vi "BMU诊断标定.vi"(8 "CAN端口":u16(ring), 9 "设备索引号":u16(ring), 10 "CAN卡类型":u32(ring)=21) -> ()   [LabVIEW 2013] (continued)
              n52 = call <vilib>:"Get Key Names.vi"("section"=w374, "refnum"=w373) -> ("key names"=w175:string[], "refnum out"=w375:T19)  [unwired: 6 in, 2 out]
              n53 = for {
                tunnel: w375 -> [w387]
                tunnel: w374 -> [w386]
                tunnel: w175 -> [w385] mode=indexing
                tunnel: [w384] -> w174 mode=indexing
                n54 = call-poly <vilib>:"Read Key.vi"("section"=w386, "key"=w385, "refnum"=w387) -> ("value"=w384:string)  [unwired: 5 in, 3 out]
              }
              n55 = Search 1D Array(1D array=w175, element="总电压过高一级" ("元素"), start index (0)=0 ("开始索引(0)")) -> (index of element=w255:i32)
              n56 = Search 1D Array(1D array=w175, element="风机开启温度" ("元素"), start index (0)=w255) -> (index of element=w246:i32)
              n57 = Search 1D Array(1D array=w175, element="电池串联" ("元素"), start index (0)=w246) -> (index of element=w244:i32)
              n58 = Decrement(x=w255) -> (x-1=w372:i32)
              n59 = Array Subset(array=w175, index=1 ("索引"), length=w372) -> (w220:string[])
              n60 = Array Subset(array=w174, index=1 ("索引"), length=w372) -> (w217:string[])
              n61 = Delete From Array(array=w217, length=7 ("长度"), index=0 ("索引")) -> (deleted portion=w214:string[], array with subset deleted=w164:string[])
              n62 = Delete From Array(array=w220, length=7 ("长度"), index=0 ("索引")) -> (array with subset deleted=w173:string[])  [unwired: 1 out]
              n63 = Search 1D Array(1D array=w175, element="分流器型号" ("元素")) -> (index of element=w178:i32)  [unwired: 1 in]
              n64 = Index Array(array=w174, index=0 ("索引")) -> (element=w348:string)
              n65 = Decimal String To Number(string=w348) -> (number=w165:i32)  [unwired: 2 in, 1 out]
              n66 = Search 1D Array(1D array=w173, element="主板电池节数" ("元素")) -> (index of element=w339:i32)  [unwired: 1 in]
              n67 = Search 1D Array(1D array=w173, element="主板温度起始值" ("元素")) -> (index of element=w336:i32)  [unwired: 1 in]
              n68 = Search 1D Array(1D array=w173, element="第一个保险通道" ("元素")) -> (index of element=w335:i32)  [unwired: 1 in]
              n69 = Search 1D Array(1D array=w173, element="主板温度个数" ("元素")) -> (index of element=w337:i32)  [unwired: 1 in]
              n70 = Search 1D Array(1D array=w173, element="主板电压起始值" ("元素")) -> (index of element=w338:i32)  [unwired: 1 in]
              n71 = Search 1D Array(1D array=w173, element="第1通道电压个数" ("元素")) -> (index of element=w334:i32)  [unwired: 1 in]
              n72 = Index Array(array=w174, index=w178) -> (element=w177:string)
              n73 = for {
                N: 4 -> [_]
                tunnel: w214 -> [w383] mode=indexing
                tunnel: [w382] -> w363 mode=indexing
                n74 = Fract/Exp String To Number(string=w383) -> (number=w382:dbl)  [unwired: 3 in, 1 out]
              }
              n75 = Increment(x=w165) -> (x+1=w347:i32)
              n76 = Increment(x=w165) -> (x+1=w332:i32)
              n77 = Increment(x=w165) -> (x+1=w345:i32)
              n78 = Increment(x=w165) -> (x+1=w346:i32)
              n79 = global write "读配置文件全局.vi" "从板个数"(w165) -> ()
              n80 = local write "从板个数"(w165) -> ()
              n81 = Decimal String To Number(string=w177) -> (number=w176:i32)  [unwired: 2 in, 1 out]
              n82 = Index Array(array=w214, index #1=4 ("索引"), index #2=5 ("索引"), index #3=6 ("索引")) -> (element #1=w354:string, element #2=w353:string, element #3=w352:string)
              n83 = Index Array(array=w363) -> (element #1=w361:dbl, element #2=w360:dbl, element #3=w359:dbl, element #4=w358:dbl)  [unwired: 4 in]
              n84 = global write "EV05全局变量1.vi" "分流器型号"(w176) -> ()
              n85 = Array Subset(array=w164, index=w339, length=w347) -> (w331:string[])
              n86 = Array Subset(array=w164, index=w338, length=w346) -> (w329:string[])
              n87 = Array Subset(array=w164, index=w337, length=w345) -> (w328:string[])
              n88 = Array Subset(array=w164, index=w336, length=w332) -> (w327:string[])
              n89 = Array Subset(array=w164, index=w335, length=20 ("长度")) -> (w326:string[])
              n90 = Array Subset(array=w164, index=w334, length=w333) -> (w330:string[])
              n91 = Multiply(x=w165, y=2) -> (x*y=w166:i32)
              n92 = control-ref of="项目信息2"() -> (w366:refnum<vi>)
              n93 = Array Subset(array=w164, index=0 ("索引"), length=w166) -> (w163:string[])
              n94 = Insert Into Array(array=w331, new element #1=w330, new element #2=w329, new element #3=w328, new element #4=w327, new element #5=w326) -> ()  [unwired: 1 in, 1 out]
              n95 = property class="Clust (严格)"(reference=w366) -> (reference out=w364:refnum<vi>, "Value"=w365:T9)  [unwired: 1 in, 1 out]
              n96 = Multiply(x=w165, y=2) -> (x*y=w170:i32)
              n97 = Array Subset(array=w173, index=w339, length=w332) -> (w204:string[])
              n98 = Array Subset(array=w173, index=w338, length=w332) -> (w202:string[])
              n99 = Array Subset(array=w173, index=w337, length=w332) -> (w201:string[])
              n100 = Array Subset(array=w173, index=w336) -> (w200:string[])  [unwired: 1 in]
              n101 = Array Subset(array=w173, index=w335, length=w333) -> (w199:string[])
              n102 = Array Subset(array=w173, index=w334, length=w333) -> (w203:string[])
              n103 = Array Subset(array=w173, index=0 ("索引"), length=w170) -> (w169:string[])
              n104 = global write "读配置文件全局.vi" "表格输入"(w163) -> ()
              n105 = Build Array(w169, w163) -> (w325:string[][])
              n106 = Bundle(cluster=w365, "电池额定容量(A)"=w361, "使用者"=w351, "电池实际容量(A)"=w360, "车架(牌)号"=w353, "配置文件版本"=w352, "SOH(%)"=w358, "SOC(%)"=w359, "产品编号"=w354) -> (w191:T9)  [unwired: 1 in]
              n107 = Transpose 2D Array(2D array=w325) -> (transposed array=w192:string[][])
              n108 = Multiply(x=w165, y=4) -> (x*y=w196:i32)
              n109 = Insert Into Array(array=w204, new element #1=w203, new element #2=w202, new element #3=w201, new element #4=w200, new element #5=w199) -> (w198:string[])  [unwired: 1 in]
              n110 = Add(x=w196, y=44) -> (x+y=w194:i32)
              n111 = local write "项目信息"(w192) -> ()
              n112 = property class="Clust (严格)"(reference=w364, "Value"=w191) -> ()  [unwired: 1 in, 2 out]
              n113 = global write "读配置文件全局.vi" "项目信息"(w191) -> ()
              n114 = Array Subset(array=w174, index=w244, length=15 ("长度")) -> (w182:string[])
              n115 = Array Subset(array=w198, index=0 ("索引"), length=w194) -> ()  [unwired: 1 out]
              n116 = Array Subset(array=w174, index=w246, length=15 ("长度")) -> (w251:string[])
              n117 = Delete From Array(array=w182, length=4 ("长度"), index=6 ("索引")) -> (deleted portion=w238:string[], array with subset deleted=w237:string[])
              n118 = for {
                tunnel: w251 -> [w379] mode=indexing
                tunnel: [w378] -> w250 mode=indexing
                n119 = Fract/Exp String To Number(string=w379) -> (number=w378:dbl)  [unwired: 3 in, 1 out]
              }
              n120 = for {
                tunnel: w237 -> [w377] mode=indexing
                tunnel: [w376] -> w236 mode=indexing
                n121 = Fract/Exp String To Number(string=w377) -> (number=w376:dbl)  [unwired: 3 in, 1 out]
              }
              n122 = Array Subset(array=w174, index=w255, length=51 ("长度")) -> (w324:string[])
              n123 = for {
                tunnel: w324 -> [w381] mode=indexing
                tunnel: [w380] -> w323 mode=indexing
                n124 = Fract/Exp String To Number(string=w381) -> (number=w380:dbl)  [unwired: 3 in, 1 out]
              }
              n125 = Index Array(array=w236) -> (element #1=w231:dbl, element #2=w230:dbl, element #3=w229:dbl, element #4=w228:dbl, element #5=w227:dbl, element #6=w226:dbl, element #7=w225:dbl, element #8=w224:dbl, element #9=w223:dbl, element #10=w222:dbl, element #11=w221:dbl)  [unwired: 11 in]
              n126 = Delete From Array(array=w250, length=7 ("长度"), index=0 ("索引")) -> (deleted portion=w187:dbl[], array with subset deleted=w248:dbl[])
              n127 = Delete From Array(array=w323, length=17 ("长度"), index=0 ("索引")) -> (deleted portion=w184:dbl[], array with subset deleted=w320:dbl[])
              n128 = Array To Cluster(array=w187) -> (cluster=w249:T20)
              n129 = global write "读配置文件全局.vi" "加热控制参数"(w187) -> ()
              n130 = Index Array(array=w248) -> (element #1=w212:dbl, element #2=w211:dbl, element #3=w210:dbl, element #4=w209:dbl, element #5=w208:dbl, element #6=w207:dbl, element #7=w206:dbl, element #8=w205:dbl)  [unwired: 8 in]
              n131 = Delete From Array(array=w320, length=17 ("长度"), index=0 ("索引")) -> (deleted portion=w183:dbl[], array with subset deleted=w180:dbl[])
              n132 = Index Array(array=w238) -> (element #1=w235:string, element #2=w234:string, element #3=w232:string, element #4=w233:string)  [unwired: 4 in]
              n133 = local write "加热控制参数"(w249) -> ()
              n134 = global write "读配置文件全局.vi" "一级故障"(w184) -> ()
              n135 = local read "一级故障 5"() -> (w213:T12)
              n136 = control-ref of="电池信息"() -> (w242:refnum<vi>)
              n137 = global write "读配置文件全局.vi" "二级故障"(w183) -> ()
              n138 = global write "读配置文件全局.vi" "三级故障"(w180) -> ()
              n139 = Bundle(cluster=w213, "最大允许单体电压"=w212, "最大允许总电压"=w208, "最小允许单体电压"=w211, "最大允许充电电流"=w210, "最小允许充电电流"=w209, "最大允许充电温度"=w207, "最小允许充电温度"=w206, "电流步长"=w205) -> (w186:T12)
              n140 = property class="Clust (严格)"(reference=w242) -> (reference out=w243:refnum<vi>, "Value"=w241:T13)  [unwired: 1 in, 1 out]
              n141 = Bundle(cluster=w241, "电池串联"=w231, "电池并联"=w230, "累计放电总安时"=w224, "电池包额定容量"=w229, "电池包额定能量(kWh)"=w228, "电池包额定总电压"=w227, "累计充电总安时"=w225, "电池充满次数"=w222, "电池放空次数"=w223, "电池充电次数"=w221, "电池生产日期"=w232, "电池厂家"=w235, "电池类型"=w234, "电池包组号"=w233, "实际容量"=w226) -> (w181:T13)  [unwired: 2 in]
              n142 = Cluster To Array(cluster=w186) -> (array=w185:dbl[])
              n143 = local write "一级故障 5"(w186) -> ()
              n144 = global write "读配置文件全局.vi" "充电控制参数"(w185) -> ()
              n145 = Index Array(array=w184) -> (element #1=w313:dbl, element #2=w312:dbl, element #3=w311:dbl, element #4=w310:dbl, element #5=w309:dbl, element #6=w308:dbl, element #7=w307:dbl, element #8=w306:dbl, element #9=w305:dbl, element #10=w304:dbl, element #11=w303:dbl, element #12=w302:dbl, element #13=w301:dbl, element #14=w300:dbl, element #15=w299:dbl, element #16=w298:dbl, element #17=w297:dbl)  [unwired: 17 in]
              n146 = global write "读配置文件全局.vi" "电池信息"(w181) -> ()
              n147 = Index Array(array=w183) -> (element #1=w280:dbl, element #2=w281:dbl, element #3=w282:dbl, element #4=w283:dbl, element #5=w284:dbl, element #6=w285:dbl, element #7=w286:dbl, element #8=w287:dbl, element #9=w288:dbl, element #10=w289:dbl, element #11=w290:dbl, element #12=w291:dbl, element #13=w292:dbl, element #14=w293:dbl, element #15=w294:dbl, element #16=w295:dbl, element #17=w296:dbl)  [unwired: 17 in]
              n148 = Index Array(array=w180) -> (element #1=w275:dbl, element #2=w274:dbl, element #3=w273:dbl, element #4=w272:dbl, element #5=w271:dbl, element #6=w270:dbl, element #7=w269:dbl, element #8=w268:dbl, element #9=w267:dbl, element #10=w266:dbl, element #11=w265:dbl, element #12=w264:dbl, element #13=w263:dbl, element #14=w262:dbl, element #15=w261:dbl, element #16=w260:dbl, element #17=w259:dbl)  [unwired: 17 in]
              n149 = control-ref of="一级故障 3"() -> (w258:refnum<vi>)
              n150 = control-ref of="一级故障 2"() -> (w277:refnum<vi>)
              n151 = property class="Clust (严格)"(reference=w277) -> (reference out=w279:refnum<vi>, "Value"=w278:T10)  [unwired: 1 in, 1 out]
              n152 = property class="Clust (严格)"(reference=w258) -> (reference out=w257:refnum<vi>, "Value"=w276:T10)  [unwired: 1 in, 1 out]
              n153 = property class="Clust (严格)"(reference=w243, "Value"=w181) -> ()  [unwired: 1 in, 2 out]
              n154 = Bundle(cluster=w278, "总电压过高"=w280, "整组电压不均衡"=w284, "SOC过高"=w292, "单体电压过高"=w288, "总电压过低"=w281, "温度过高"=w282, "温度过低"=w283, "单组电压不均衡"=w285, "整组温度不均衡"=w286, "单组温度不均衡"=w287, "单体电压过低"=w289, "充电电流过高"=w290, "放电电流过高"=w291, "SOC过低"=w293, "内阻过大"=w294, "极柱温度过高"=w295, "SOH过低"=w296) -> (w189:T10)
              n155 = Bundle(cluster=w276, "总电压过高"=w275, "整组电压不均衡"=w271, "SOC过高"=w263, "单体电压过高"=w267, "总电压过低"=w274, "温度过高"=w273, "温度过低"=w272, "单组电压不均衡"=w270, "整组温度不均衡"=w269, "单组温度不均衡"=w268, "单体电压过低"=w266, "充电电流过高"=w265, "放电电流过高"=w264, "SOC过低"=w262, "内阻过大"=w261, "极柱温度过高"=w260, "SOH过低"=w259) -> (w188:T10)
              n156 = control-ref of="一级故障"() -> (w316:refnum<vi>)
              n157 = property class="Clust (严格)"(reference=w316) -> (reference out=w314:refnum<vi>, "Value"=w315:T10)  [unwired: 1 in, 1 out]
              n158 = Bundle(cluster=w315, "总电压过高"=w313, "整组电压不均衡"=w309, "SOC过高"=w301, "单体电压过高"=w305, "总电压过低"=w312, "温度过高"=w311, "温度过低"=w310, "单组电压不均衡"=w308, "整组温度不均衡"=w307, "单组温度不均衡"=w306, "单体电压过低"=w304, "充电电流过高"=w303, "放电电流过高"=w302, "SOC过低"=w300, "内阻过大"=w299, "极柱温度过高"=w298, "SOH过低"=w297) -> (w190:T10)
              n159 = property class="Clust (严格)"(reference=w314, "Value"=w190) -> ()  [unwired: 1 in, 2 out]
              n160 = property class="Clust (严格)"(reference=w279, "Value"=w189) -> ()  [unwired: 1 in, 2 out]
              n161 = property class="Clust (严格)"(reference=w257, "Value"=w188) -> ()  [unwired: 1 in, 2 out]
            }
            frame #2 {
              w452 = 1 ("索引")
              # "均衡计算-电压高阀值1级"
              n162 = call <vilib>:"Get Section Names.vi"("refnum"=w467) -> ("section names"=w468:string[], "refnum out"=w472:T19)  [unwired: 8 in, 1 out]
              n163 = Delete From Array(array=w468, length=2 ("长度"), index=0 ("索引")) -> (array with subset deleted=w471:string[])  [unwired: 1 out]
              n164 = for {
                tunnel: w471 -> [w488] mode=indexing
                tunnel: w472 -> [w489]
                tunnel: [w481] -> w450 mode=indexing
                tunnel: [w480] -> w394
                n165 = call <vilib>:"Get Key Names.vi"("section"=w488, "refnum"=w489) -> ("key names"=w480:string[], "refnum out"=w487:T19)  [unwired: 6 in, 2 out]
                n166 = for {
                  tunnel: w480 -> [w493] mode=indexing
                  tunnel: w488 -> [w492]
                  tunnel: w487 -> [w491]
                  tunnel: [w490] -> w481 mode=indexing
                  n167 = call-poly <vilib>:"Read Key.vi"("section"=w492, "key"=w493, "refnum"=w491) -> ("value"=w490:string)  [unwired: 5 in, 3 out]
                }
                n168 = Index Array(array=w481, index=0 ("索引")) -> (element=w484:string)
                n169 = local read "输出数组"() -> (w485:string[][])
                n170 = Decimal String To Number(string=w484) -> (number=w483:i32)  [unwired: 2 in, 1 out]
                n171 = Decrement(x=w483) -> (x-1=w479:i32)
                n172 = Replace Array Subset(array=w485, new element=w481, index (col)=w479) -> (w482:string[][])  [unwired: 1 in]
                n173 = local write "输出数组"(w482) -> ()
              }
              "key names" <- w394
              n174 = Decrement(x=w388) -> (x-1=w466:i32)
              n175 = Index Array(array=w450, index (row)=w466) -> (element=w393:string[])  [unwired: 1 in]
              n176 = Search 1D Array(1D array=w394, element="风机开启温度" ("元素")) -> (index of element=w455:i32)  [unwired: 1 in]
              n177 = Search 1D Array(1D array=w394, element="电压过高一级" ("元素"), start index (0)=w455) -> (index of element=w419:i32)
              n178 = Search 1D Array(1D array=w394, element="均衡计算-电压高阀值1级" ("元素"), start index (0)=w419) -> (index of element=w417:i32)
              n179 = Array Subset(array=w393, index=w417, length=17 ("长度")) -> (w416:string[])
              n180 = Decrement(x=w455) -> (x-1=w453:i32)
              n181 = Array Subset(array=w393, index=w452, length=w453) -> (w391:string[])
              n182 = Array Subset(array=w393, index=w419, length=21 ("长度")) -> (w464:string[])
              n183 = Array Subset(array=w394, index=w452, length=w453) -> (w430:string[])
              n184 = Index Array(array=w393, index=0 ("索引")) -> (element=w425:string)
              n185 = Array Subset(array=w393, index=w455, length=7 ("长度")) -> (w458:string[])
              n186 = for {
                tunnel: w416 -> [w474] mode=indexing
                tunnel: [w473] -> w415 mode=indexing
                n187 = Fract/Exp String To Number(string=w474) -> (number=w473:dbl)  [unwired: 3 in, 1 out]
              }
              n188 = for {
                tunnel: w464 -> [w476] mode=indexing
                tunnel: [w475] -> w465 mode=indexing
                n189 = Fract/Exp String To Number(string=w476) -> (number=w475:dbl)  [unwired: 3 in, 1 out]
              }
              n190 = Decimal String To Number(string=w425) -> (number=w424:i32)  [unwired: 2 in, 1 out]
              n191 = for {
                tunnel: w458 -> [w478] mode=indexing
                tunnel: [w477] -> w427 mode=indexing
                n192 = Fract/Exp String To Number(string=w478) -> (number=w477:dbl)  [unwired: 3 in, 1 out]
              }
              n193 = global write "读配置文件全局2.vi" "从板板号"(w424) -> ()
              n194 = Delete From Array(array=w465, length=7 ("长度"), index=0 ("索引")) -> (deleted portion=w429:dbl[], array with subset deleted=w461:dbl[])
              n195 = Array To Cluster(array=w427) -> (cluster=w449:T20)
              n196 = global write "读配置文件全局2.vi" "加热控制参数"(w427) -> ()
              n197 = Delete From Array(array=w461, length=7 ("长度"), index=0 ("索引")) -> (deleted portion=w422:dbl[], array with subset deleted=w423:dbl[])
              n198 = local write "加热控制参数"(w449) -> ()
              n199 = Array To Cluster(array=w429) -> (cluster=w433:T20)
              n200 = Array To Cluster(array=w423) -> (cluster=w431:T20)
              n201 = Array To Cluster(array=w422) -> (cluster=w432:T20)
              n202 = local write "从板号"(w388) -> ()
              n203 = global write "读配置文件全局2.vi" "三级故障阀值"(w423) -> ()
              n204 = global write "读配置文件全局2.vi" "一级故障阀值"(w429) -> ()
              n205 = global write "读配置文件全局2.vi" "二级故障阀值"(w422) -> ()
              n206 = local write "一级故障 6"(w433) -> ()
              n207 = local write "一级故障 8"(w431) -> ()
              n208 = local write "一级故障 7"(w432) -> ()
              n209 = Search 1D Array(1D array=w430, element="第1通道电压个数" ("元素")) -> (index of element=w441:i32)  [unwired: 1 in]
              n210 = Search 1D Array(1D array=w430, element="电压个数" ("元素")) -> ()  [unwired: 1 in, 1 out]
              n211 = Search 1D Array(1D array=w430, element="温度个数" ("元素")) -> (index of element=w443:i32)  [unwired: 1 in]
              n212 = Search 1D Array(1D array=w430, element="第一个保险通道" ("元素")) -> (index of element=w442:i32)  [unwired: 1 in]
              n213 = Array Subset(array=w391, length=2 ("长度")) -> (w438:string[])  [unwired: 1 in]
              n214 = Array Subset(array=w391, index=w443, length=2 ("长度")) -> (w436:string[])
              n215 = Array Subset(array=w391, index=w442, length=20 ("长度")) -> (w435:string[])
              n216 = Array Subset(array=w391, index=w441, length=20 ("长度")) -> (w437:string[])
              n217 = Array Subset(array=w391, length=27 ("长度")) -> (w390:string[])  [unwired: 1 in]
              n218 = Insert Into Array(array=w438, new element #1=w437, new element #2=w436, new element #3=w435) -> ()  [unwired: 1 in, 1 out]
              n219 = Build Array(string[] ["电压个数", "温度个数", "第一个保险通道", "第一个保险位置", "第二个保险通道", "第二个保险位置", "第三个保险通道", "第三个保险位置", "第四个保险通道", "第四个保险位置", "第五个保险通道", "第五个保险位置", "第六个保险通道", "第六个保险位置", "第七个保险通道", "第七个保险位置", "第八个保险通道", "第八个保险位置", "第九个保险通道", "第九个保险位置", "第十个保险通道", "第十个保险位置", "第1通道电压个数", "第2通道电压个数", "第3通道电压个数", "第4通道电压个数", "第5通道电压个数"], w390) -> (w434:string[][])
              n220 = global write "读配置文件全局2.vi" "表格"(w390) -> ()
              n221 = Index Array(array=w415) -> (element #1=w412:dbl, element #2=w411:dbl, element #3=w410:dbl, element #4=w409:dbl, element #5=w408:dbl, element #6=w407:dbl, element #7=w406:dbl, element #8=w405:dbl, element #9=w404:dbl, element #10=w403:dbl, element #11=w402:dbl, element #12=w401:dbl, element #13=w400:dbl, element #14=w399:dbl, element #15=w398:dbl, element #16=w397:dbl, element #17=w396:dbl, element #18=w395:dbl)  [unwired: 18 in]
              n222 = Transpose 2D Array(2D array=w434) -> (transposed array=w428:string[][])
              n223 = local write "项目信息 2"(w428) -> ()
              n224 = local read "均衡参数"() -> (w414:T17)
              n225 = Bundle(cluster=w414, "充电结束电压(90%)"=w405, "充电结束电压(91%)"=w404, "充电结束电压(92%)"=w403, "充电结束电压(93%)"=w402, "充电结束电压(94%)"=w401, "均衡计算-电压高阀值1级"=w412, "均衡计算-电压高阀值2级"=w411, "均衡计算-电压低阀值1级"=w410, "均衡计算-电压低阀值2级"=w409, "均衡计算-最低电压阀值"=w408, "均衡停止-最低电压阀值"=w407, "均衡计算-电压极差阀值"=w406, "充电结束电压(95%)"=w400, "充电结束电压(96%)"=w399, "充电结束电压(97%)"=w398, "充电结束电压(98%)"=w397, "充电结束电压(99%)"=w396, "充电结束电压(100%)"=w395) -> (w413:T17)
              n226 = local write "均衡参数"(w413) -> ()
            }
            frame #3 {
              n227 = Build Array("读取完成") -> (w497:string[])
              n228 = property on="全部写入" class="Bool (严格)"("DisabledEnum"=0) -> ()  [unwired: 2 in, 2 out]
              n229 = call "表格编辑.vi"("新元素/子数组"=w497, "活动单元格:单元格背景色"=u32 6618880, "MCListbox引用句柄"=w494) -> ()  [unwired: 9 out]
            }
          }
        }
      }
    }
  }
  n230 = local write "项目信息 2"(string[][] [["电压个数", "36"], ["温度个数", "45"], ["第一个保险通道", "0"], ["第一个保险位置", "0"], ["第二个保险通道", "0"], ["第二个保险位置", "0"], ["第三个保险通道", "0"], ["第三个保险位置", "0"], ["第四个保险通道", "0"], ["第四个保险位置", "0"], ["第五个保险通道", "0"], ["第五个保险位置", "0"], ["第六个保险通道", "0"], ["第六个保险位置", "0"], ["第七个保险通道", "0"], ["第七个保险位置", "0"], ["第八个保险通道", "0"], ["第八个保险位置", "0"], ["第九个保险通道", "0"], ["第九个保险位置", "0"], ["第十个保险通道", "0"], ["第十个保险位置", "0"], ["第1通道电压个数", "11"], ["第2通道电压个数", "12"], ["第3通道电压个数", "12"], ["第4通道电压个数", "12"], ["第5通道电压个数", "12"]] ("项目信息 2")) -> ()
  n231 = stacked-sequence {
    frame #0 {
    }
  }
  n232 = Index Array(array=w50, index (col)=0 ("索引 (行)")) -> (element=w53:string[])  [unwired: 1 in]
  n233 = Index Array(array=w50, index (col)=1 ("禁用的索引 (列)")) -> (element=w43:string[])  [unwired: 1 in]
  n234 = local read "从板个数"() -> (w45:dbl)
  n235 = Array Subset(array=w53, index=0 ("索引"), length=w45) -> (w52:string[])
  n236 = Array Subset(array=w53, index=10 ("索引"), length=w45) -> (w51:string[])
  n237 = Array Subset(array=w43, index=0 ("索引"), length=w45) -> (w49:string[])
  n238 = Array Subset(array=w43, index=10 ("索引"), length=w45) -> (w44:string[])
  n239 = Insert Into Array(array=w52, new element=w51) -> (w42:string[])  [unwired: 1 in]
  n240 = Insert Into Array(array=w49, new element=w44) -> (w41:string[])  [unwired: 1 in]
  n241 = Build Array(w42, w41) -> (w40:string[][])
  n242 = local write "停止"(FALSE ("停止")) -> ()
  n243 = Transpose 2D Array(2D array=w40) -> (transposed array=w39:string[][])
  n244 = local write "项目信息"(w39) -> ()
  n245 = stacked-sequence {
    tunnel: [w500] -> w29
    tunnel: ["error in (no error)"] -> w28
    frame #0 {
      w502 = 1
      w503 = string[][] []
      w521 = string[] ["", "", "", "", "", "", "", "", "", "", "", "", "", "", "", "", "", "", "", "", "", "", "", "", "", "", "", "", "", "", "", ""]
      w520 = string[][] [["", "", "", "", "", "", "", "", "", "", "", "", "", "", "", "", "", "", "", "", "", "", "", "", "", "", "", "", "", "", "", "", "", "", "", "", "", "", "", "", ""], ["", "", "", "", "", "", "", "", "", "", "", "", "", "", "", "", "", "", "", "", "", "", "", "", "", "", "", "", "", "", "", "", "", "", "", "", "", "", "", "", ""], ["", "", "", "", "", "", "", "", "", "", "", "", "", "", "", "", "", "", "", "", "", "", "", "", "", "", "", "", "", "", "", "", "", "", "", "", "", "", "", "", ""], ["", "", "", "", "", "", "", "", "", "", "", "", "", "", "", "", "", "", "", "", "", "", "", "", "", "", "", "", "", "", "", "", "", "", "", "", "", "", "", "", ""], ["", "", "", "", "", "", "", "", "", "", "", "", "", "", "", "", "", "", "", "", "", "", "", "", "", "", "", "", "", "", "", "", "", "", "", "", "", "", "", "", ""], ["", "", "", "", "", "", "", "", "", "", "", "", "", "", "", "", "", "", "", "", "", "", "", "", "", "", "", "", "", "", "", "", "", "", "", "", "", "", "", "", ""], ["", "", "", "", "", "", "", "", "", "", "", "", "", "", "", "", "", "", "", "", "", "", "", "", "", "", "", "", "", "", "", "", "", "", "", "", "", "", "", "", ""], ["", "", "", "", "", "", "", "", "", "", "", "", "", "", "", "", "", "", "", "", "", "", "", "", "", "", "", "", "", "", "", "", "", "", "", "", "", "", "", "", ""], ["", "", "", "", "", "", "", "", "", "", "", "", "", "", "", "", "", "", "", "", "", "", "", "", "", "", "", "", "", "", "", "", "", "", "", "", "", "", "", "", ""], ["", "", "", "", "", "", "", "", "", "", "", "", "", "", "", "", "", "", "", "", "", "", "", "", "", "", "", "", "", "", "", "", "", "", "", "", "", "", "", "", ""], ["", "", "", "", "", "", "", "", "", "", "", "", "", "", "", "", "", "", "", "", "", "", "", "", "", "", "", "", "", "", "", "", "", "", "", "", "", "", "", "", ""], ["", "", "", "", "", "", "", "", "", "", "", "", "", "", "", "", "", "", "", "", "", "", "", "", "", "", "", "", "", "", "", "", "", "", "", "", "", "", "", "", ""], ["", "", "", "", "", "", "", "", "", "", "", "", "", "", "", "", "", "", "", "", "", "", "", "", "", "", "", "", "", "", "", "", "", "", "", "", "", "", "", "", ""], ["", "", "", "", "", "", "", "", "", "", "", "", "", "", "", "", "", "", "", "", "", "", "", "", "", "", "", "", "", "", "", "", "", "", "", "", "", "", "", "", ""], ["", "", "", "", "", "", "", "", "", "", "", "", "", "", "", "", "", "", "", "", "", "", "", "", "", "", "", "", "", "", "", "", "", "", "", "", "", "", "", "", ""], ["", "", "", "", "", "", "", "", "", "", "", "", "", "", "", "", "", "", "", "", "", "", "", "", "", "", "", "", "", "", "", "", "", "", "", "", "", "", "", "", ""], ["", "", "", "", "", "", "", "", "", "", "", "", "", "", "", "", "", "", "", "", "", "", "", "", "", "", "", "", "", "", "", "", "", "", "", "", "", "", "", "", ""], ["", "", "", "", "", "", "", "", "", "", "", "", "", "", "", "", "", "", "", "", "", "", "", "", "", "", "", "", "", "", "", "", "", "", "", "", "", "", "", "", ""], ["", "", "", "", "", "", "", "", "", "", "", "", "", "", "", "", "", "", "", "", "", "", "", "", "", "", "", "", "", "", "", "", "", "", "", "", "", "", "", "", ""], ["", "", "", "", "", "", "", "", "", "", "", "", "", "", "", "", "", "", "", "", "", "", "", "", "", "", "", "", "", "", "", "", "", "", "", "", "", "", "", "", ""], ["", "", "", "", "", "", "", "", "", "", "", "", "", "", "", "", "", "", "", "", "", "", "", "", "", "", "", "", "", "", "", "", "", "", "", "", "", "", "", "", ""], ["", "", "", "", "", "", "", "", "", "", "", "", "", "", "", "", "", "", "", "", "", "", "", "", "", "", "", "", "", "", "", "", "", "", "", "", "", "", "", "", ""], ["", "", "", "", "", "", "", "", "", "", "", "", "", "", "", "", "", "", "", "", "", "", "", "", "", "", "", "", "", "", "", "", "", "", "", "", "", "", "", "", ""], ["", "", "", "", "", "", "", "", "", "", "", "", "", "", "", "", "", "", "", "", "", "", "", "", "", "", "", "", "", "", "", "", "", "", "", "", "", "", "", "", ""], ["", "", "", "", "", "", "", "", "", "", "", "", "", "", "", "", "", "", "", "", "", "", "", "", "", "", "", "", "", "", "", "", "", "", "", "", "", "", "", "", ""], ["", "", "", "", "", "", "", "", "", "", "", "", "", "", "", "", "", "", "", "", "", "", "", "", "", "", "", "", "", "", "", "", "", "", "", "", "", "", "", "", ""], ["", "", "", "", "", "", "", "", "", "", "", "", "", "", "", "", "", "", "", "", "", "", "", "", "", "", "", "", "", "", "", "", "", "", "", "", "", "", "", "", ""], ["", "", "", "", "", "", "", "", "", "", "", "", "", "", "", "", "", "", "", "", "", "", "", "", "", "", "", "", "", "", "", "", "", "", "", "", "", "", "", "", ""], ["", "", "", "", "", "", "", "", "", "", "", "", "", "", "", "", "", "", "", "", "", "", "", "", "", "", "", "", "", "", "", "", "", "", "", "", "", "", "", "", ""], ["", "", "", "", "", "", "", "", "", "", "", "", "", "", "", "", "", "", "", "", "", "", "", "", "", "", "", "", "", "", "", "", "", "", "", "", "", "", "", "", ""], ["", "", "", "", "", "", "", "", "", "", "", "", "", "", "", "", "", "", "", "", "", "", "", "", "", "", "", "", "", "", "", "", "", "", "", "", "", "", "", "", ""], ["", "", "", "", "", "", "", "", "", "", "", "", "", "", "", "", "", "", "", "", "", "", "", "", "", "", "", "", "", "", "", "", "", "", "", "", "", "", "", "", ""], ["", "", "", "", "", "", "", "", "", "", "", "", "", "", "", "", "", "", "", "", "", "", "", "", "", "", "", "", "", "", "", "", "", "", "", "", "", "", "", "", ""], ["", "", "", "", "", "", "", "", "", "", "", "", "", "", "", "", "", "", "", "", "", "", "", "", "", "", "", "", "", "", "", "", "", "", "", "", "", "", "", "", ""], ["", "", "", "", "", "", "", "", "", "", "", "", "", "", "", "", "", "", "", "", "", "", "", "", "", "", "", "", "", "", "", "", "", "", "", "", "", "", "", "", ""], ["", "", "", "", "", "", "", "", "", "", "", "", "", "", "", "", "", "", "", "", "", "", "", "", "", "", "", "", "", "", "", "", "", "", "", "", "", "", "", "", ""], ["", "", "", "", "", "", "", "", "", "", "", "", "", "", "", "", "", "", "", "", "", "", "", "", "", "", "", "", "", "", "", "", "", "", "", "", "", "", "", "", ""], ["", "", "", "", "", "", "", "", "", "", "", "", "", "", "", "", "", "", "", "", "", "", "", "", "", "", "", "", "", "", "", "", "", "", "", "", "", "", "", "", ""], ["", "", "", "", "", "", "", "", "", "", "", "", "", "", "", "", "", "", "", "", "", "", "", "", "", "", "", "", "", "", "", "", "", "", "", "", "", "", "", "", ""], ["", "", "", "", "", "", "", "", "", "", "", "", "", "", "", "", "", "", "", "", "", "", "", "", "", "", "", "", "", "", "", "", "", "", "", "", "", "", "", "", ""], ["", "", "", "", "", "", "", "", "", "", "", "", "", "", "", "", "", "", "", "", "", "", "", "", "", "", "", "", "", "", "", "", "", "", "", "", "", "", "", "", ""]]
      w509 = TRUE
      w505 = u32 16777215
      w500 = FALSE ("判定2")
      n246 = control-ref of="结果"() -> (w506:refnum<vi>)
      n247 = control-ref of="模块软件版本 2"() -> (w507:refnum<vi>)
      n248 = control-ref of="结果"() -> (w508:refnum<vi>)
      n249 = control-ref of="单选选项2"() -> (w524:refnum<vi>)
      n250 = control-ref of="单选选项1"() -> (w525:refnum<vi>)
      n251 = local write "key names"(string[] []) -> ()
      n252 = property on="项目信息" class="Tbl (严格)"("Disabled"=w502) -> ()  [unwired: 2 in, 2 out]
      n253 = property on="电池实际容量(A)" class="DigNum (严格)"("Disabled"=w502) -> ()  [unwired: 2 in, 2 out]
      n254 = property on="使用者" class="DigNum (严格)"("Disabled"=w502) -> ()  [unwired: 2 in, 2 out]
      n255 = property on="SOH(%)" class="DigNum (严格)"("Disabled"=w502) -> ()  [unwired: 2 in, 2 out]
      n256 = property on="电池额定容量(A)" class="DigNum (严格)"("Disabled"=w502) -> ()  [unwired: 2 in, 2 out]
      n257 = local write "主从选择"(enum32{"主板", "从板"}."从板" ("主从选择")) -> ()
      n258 = property on="SOC(%)" class="DigNum (严格)"("Disabled"=w502) -> ()  [unwired: 2 in, 2 out]
      n259 = local write "等级 2"(T21."从板信息" ("等级 2")) -> ()
      n260 = local write "主板2"(T8."项目信息" ("主从板")) -> ()
      n261 = property class="MCListbox (严格)"(reference=w508, "ItemNames"=w503) -> ()  [unwired: 1 in, 2 out]
      n262 = property class="MCListbox (严格)"(reference=w507, "ItemNames"=w503) -> ()  [unwired: 1 in, 2 out]
      n263 = property class="MCListbox (严格)"(reference=w506, "ItemNames"=w503) -> ()  [unwired: 1 in, 2 out]
      n264 = property class="Bool (严格)"(reference=w524, "BoolText.TextColor"=u32 87470) -> ()  [unwired: 1 in, 2 out]
      n265 = property class="Bool (严格)"(reference=w525, "BoolText.TextColor"=w505) -> ()  [unwired: 1 in, 2 out]
      n266 = property on="从板号" class="DigNum (严格)"("NumText.BGColor"=w505) -> ()  [unwired: 2 in, 2 out]
      n267 = local write "主从板"(enum32{"单选选项2", "单选选项1"}."单选选项2" ("主从板")) -> ()
      n268 = property on="项目信息2" class="Clust (严格)"("DisabledEnum"=w502) -> ()  [unwired: 2 in, 2 out]
      n269 = property on="系统时钟" class="Str"("Disabled"=w502) -> ()  [unwired: 2 in, 2 out]
      n270 = property on="配置文件版本" class="Str"("Disabled"=w502) -> ()  [unwired: 2 in, 2 out]
      n271 = property on="车架(牌)号" class="Str"("Disabled"=w502) -> ()  [unwired: 2 in, 2 out]
      n272 = property on="产品编号" class="Str"("Disabled"=w502) -> ()  [unwired: 2 in, 2 out]
      n273 = local write "判定3"(w509) -> ()
      n274 = local write "清BUFF"(w509) -> ()
      n275 = local write "1"(w509) -> ()
      n276 = property on="从板个数" class="DigNum (严格)"("Visible"=w509) -> ()  [unwired: 2 in, 2 out]
      n277 = property on="从板个数" class="DigNum (严格)"("NumText.BGColor"=u32 16448250) -> ()  [unwired: 2 in, 2 out]
      n278 = Not(x=w509) -> (.not. x?=w528:bool)
      n279 = local write "布尔"(w509) -> ()
      n280 = property on="主板选项" class="Tree (严格)"("Visible"=w509) -> ()  [unwired: 2 in, 2 out]
      n281 = property on="全部写入" class="Bool (严格)"("DisabledEnum"=2) -> ()  [unwired: 2 in, 2 out]
      n282 = property on="从板选项" class="Tree (严格)"("Visible"=w528) -> ()  [unwired: 2 in, 2 out]
      n283 = property on="当前从板板号" class="DigNum (严格)"("Visible"=w528) -> ()  [unwired: 2 in, 2 out]
      n284 = control-ref of="结果"() -> (w515:refnum<vi>)
      n285 = control-ref of="结果"() -> (w512:refnum<vi>)
      n286 = local write "强制停止版本读取"(w500) -> ()
      n287 = local write "强制终止读写标记"(w500) -> ()
      n288 = control-ref of="项目信息"() -> (w513:refnum<vi>)
      n289 = local write "判定2"(w500) -> ()
      n290 = local write "停止"(w500) -> ()
      n291 = local write "控制1"(w500) -> ()
      n292 = local write "消除"(w500) -> ()
      n293 = global write "EV05全局变量1.vi" "授权功能"(w500) -> ()
      n294 = local write "继电器超时处理"(w500) -> ()
      n295 = local write "1 6"(w500) -> ()
      n296 = local write "1 7"(w500) -> ()
      n297 = local write "1 8"(w500) -> ()
      n298 = local write "1 9"(w500) -> ()
      n299 = local write "1 10"(w500) -> ()
      n300 = local write "1 2"(w500) -> ()
      n301 = local write "1 3"(w500) -> ()
      n302 = local write "1 4"(w500) -> ()
      n303 = local write "1 5"(w500) -> ()
      n304 = local write "1 11"(w500) -> ()
      n305 = for {
        N: 150 -> [_]
        tunnel: w515 -> [w538]
        i -> [w536]
        n306 = Bundle(w536, 0) -> (w534:cluster{i32, i32})  [unwired: 1 out]
        n307 = property class="MCListbox (严格)"(reference=w538, "ActiveCell"=w534, "CellBG"=u32 16448250) -> ()  [unwired: 1 in, 2 out]
      }
      n308 = for {
        N: 150 -> [_]
        tunnel: w513 -> [w533]
        i -> [w532]
        n309 = Bundle(w532, 0) -> (w530:cluster{i32, i32})  [unwired: 1 out]
        n310 = property class="Tbl (严格)"(reference=w533, "Active Cell"=w530, "Cell BG Color"=u32 16448250) -> ()  [unwired: 1 in, 2 out]
      }
      n311 = for {
        N: 150 -> [_]
        tunnel: w512 -> [w543]
        i -> [w541]
        n312 = Bundle(w541, 0) -> (w539:cluster{i32, i32})  [unwired: 1 out]
        n313 = property class="MCListbox (严格)"(reference=w543, "ActiveCell"=w539, "CellBG"=u32 16448250) -> ()  [unwired: 1 in, 2 out]
      }
      n314 = local write "加热继电器(从)"(w500) -> ()
      n315 = local write "风机继电器(从)"(w500) -> ()
      n316 = local write "DO1"(w500) -> ()
      n317 = local write "DO2"(w500) -> ()
      n318 = local write "DO1 2"(w500) -> ()
      n319 = local write "正级继电器"(w500) -> ()
      n320 = local write "负级继电器"(w500) -> ()
      n321 = local write "加热继电器"(w500) -> ()
      n322 = local write "充电继电器"(w500) -> ()
      n323 = local write "风机继电器"(w500) -> ()
      n324 = local write "预充电继电器"(w500) -> ()
      n325 = property on="保存版本信息" class="Bool (严格)"("Visible"=w500) -> ()  [unwired: 2 in, 2 out]
      n326 = property on="单个读取" class="Bool (严格)"("Visible"=w500) -> ()  [unwired: 2 in, 2 out]
      n327 = property on="单个写入" class="Bool (严格)"("Visible"=w500) -> ()  [unwired: 2 in, 2 out]
      n328 = local write "正级继电器 12"(w500) -> ()
      n329 = local write "正级继电器 2"(w500) -> ()
      n330 = local write "正级继电器 3"(w500) -> ()
      n331 = local write "正级继电器 4"(w500) -> ()
      n332 = local write "正级继电器 5"(w500) -> ()
      n333 = local write "正级继电器 6"(w500) -> ()
      n334 = local write "正级继电器 7"(w500) -> ()
      n335 = local write "正级继电器 8"(w500) -> ()
      n336 = local write "正级继电器 9"(w500) -> ()
      n337 = local write "正级继电器 10"(w500) -> ()
      n338 = local write "正级继电器 11"(w500) -> ()
      n339 = property on="从板号" class="DigNum (严格)"("Visible"=TRUE ("可见")) -> ()  [unwired: 2 in, 2 out]
      "电池故障" <- w503
      "模块版本值" <- w520
      "硬件版本" <- w521
      "模块版本名称" <- w520
      "平台软件版本" <- w521
      "项目软件版本" <- w521
      "模块个数" <- u8[] [0, 0, 0, 0, 0, 0, 0, 0, 0, 0, 0, 0, 0, 0, 0, 0, 0, 0, 0, 0, 0, 0, 0, 0, 0, 0, 0, 0, 0, 0, 0, 0] ("模块个数")
    }
  }
  n340 = stacked-sequence {
    tunnel: [w544] -> w22
    frame #0 {
      n341 = disable-structure shown="禁用" {
        frame Disabled {
          n342 = control-ref of="主板选项"() -> (w663:refnum<vi>)
          n343 = stacked-sequence {
            tunnel: w663 -> [w665 w823 w861]
            frame #0 {
              # "加热和充电控制参数"
              n344 = global read "功能码全局.vi" "主板控制类信息10"() -> (w675:bool[])
              n345 = Index Array(array=w675) -> (element #5=w669:bool, element #6=w667:bool, element #7=w668:bool, element #8=w666:bool)  [unwired: 8 in, 4 out]
              n346 = Not Or(1:w668, 2:w669) -> (0:w674:bool)
              n347 = Not Or(1:w666, 2:w667) -> (0:w672:bool)
              n348 = for {
                N: 8 -> [_]
                tunnel: w665 -> [w795]
                tunnel: w674 -> [w791]
                tunnel: [w790] -> w673
                i -> [w793]
                n349 = Add(x=w793, y=69) -> (x+y=w794:i32)
                n350 = property class="Tree (严格)"(reference=w795, "Active Item Row Number"=w794, "Disabled?"=w791) -> (error out=w790:errorcluster)  [unwired: 1 in, 1 out]
              }
              n351 = for {
                N: 9 -> [_]
                tunnel: w665 -> [w789]
                tunnel: w672 -> [w785]
                tunnel: w673 -> [w784]
                tunnel: [w783] -> w664
                i -> [w787]
                n352 = Add(x=w787, y=77) -> (x+y=w788:i32)
                n353 = property class="Tree (严格)"(reference=w789, error in=w784, "Active Item Row Number"=w788, "Disabled?"=w785) -> (error out=w783:errorcluster)  [unwired: 1 out]
              }
              n354 = stacked-sequence {
                tunnel: w665 -> [w695 _ _]
                tunnel: w664 -> [w694 _ _]
                frame #0 {
                  # "电池信息"
                  n355 = global read "功能码全局.vi" "主板版本号11"() -> (w696:bool[])
                  n356 = global read "功能码全局.vi" "主板项目信息4"() -> (w678:bool[])
                  n357 = Index Array(array=w696) -> (element #1=w692:bool, element #2=w691:bool, element #3=w685:bool, element #4=w679:bool, element #6=w684:bool, element #7=w683:bool, element #8=w682:bool)  [unwired: 8 in, 1 out]
                  n358 = Index Array(array=w678, index=4 ("索引")) -> (element=w676:bool)
                  n359 = Or(x=w685, y=w679) -> (x .or. y?=w680:bool)
                  n360 = Not(x=w683) -> (.not. x?=w687:bool)
                  n361 = Not(x=w682) -> (.not. x?=w686:bool)
                  n362 = Not(x=w684) -> (.not. x?=w688:bool)
                  n363 = property on="硬件版本号" class="Str"("Visible"=w685) -> ()  [unwired: 2 in, 2 out]
                  n364 = property on="读硬件版本号" class="Bool (严格)"("Visible"=w685) -> ()  [unwired: 2 in, 2 out]
                  n365 = property on="项目软件版本号" class="Str"("Visible"=w685) -> ()  [unwired: 2 in, 2 out]
                  n366 = property on="项目软本读取" class="Bool (严格)"("Visible"=w685) -> ()  [unwired: 2 in, 2 out]
                  n367 = property on="继电器屏1 2" class="TabCtl (严格)"("Visible"=w688) -> ()  [unwired: 2 in, 2 out]
                  n368 = property on="均衡屏" class="TabCtl (严格)"("Visible"=w686) -> ()  [unwired: 2 in, 2 out]
                  n369 = property on="继电器屏1 2" class="TabCtl (严格)"("Visible"=w688) -> ()  [unwired: 2 in, 2 out]
                  n370 = property on="DO屏" class="TabCtl (严格)"("Visible"=w687) -> ()  [unwired: 2 in, 2 out]
                  n371 = Compound Arithmetic op=OR(w684, w683, w682) -> (w681:bool)
                  n372 = Not Or(1:w691, 2:w692) -> (0:w690:bool)
                  n373 = stacked-sequence {
                    tunnel: w681 -> [_ w701 _]
                    tunnel: w680 -> [_ _ w705]
                    tunnel: w676 -> [w697 _ _]
                    frame #0 {
                      n374 = case shown="真" w697 {
                        frame False {
                        }
                        frame True {
                          n375 = local write "主界面选项"(enum32{"单选选项1", "单选选项2", "单选选项2 2", "单选选项2 3"}."单选选项2 3" ("主界面选项")) -> ()
                          n376 = local write "面板选择"(T7."高压板校正" ("面板选择")) -> ()
                        }
                      }
                      n377 = control-ref of="单选选项2 3"() -> (w698:refnum<vi>)
                      n378 = property class="Bool (严格)"(reference=w698, "Visible"=w697) -> ()  [unwired: 1 in, 2 out]
                    }
                    frame #1 {
                      n379 = control-ref of="单选选项2 2"() -> (w702:refnum<vi>)
                      n380 = case shown="真" w701 {
                        frame False {
                        }
                        frame True {
                          n381 = local write "主界面选项"(enum32{"单选选项1", "单选选项2", "单选选项2 2", "单选选项2 3"}."单选选项2 2" ("主界面选项")) -> ()
                          n382 = local write "面板选择"(enum32{"读写参数", "版本读取", "其它诊断"}."其它诊断" ("选项卡控件 2")) -> ()
                        }
                      }
                      n383 = property class="Bool (严格)"(reference=w702, "Visible"=w701) -> ()  [unwired: 1 in, 2 out]
                    }
                    frame #2 {
                      n384 = control-ref of="单选选项2"() -> (w706:refnum<vi>)
                      n385 = case shown="真" w705 {
                        frame False {
                        }
                        frame True {
                          n386 = local write "主界面选项"(enum32{"单选选项1", "单选选项2", "单选选项2 2", "单选选项2 3"}."单选选项2" ("主界面选项")) -> ()
                          n387 = local write "面板选择"(enum32{"读写参数", "版本读取", "其它诊断"}."版本读取" ("选项卡控件 2")) -> ()
                        }
                      }
                      n388 = property class="Bool (严格)"(reference=w706, "Visible"=w705) -> ()  [unwired: 1 in, 2 out]
                    }
                  }
                  n389 = for {
                    N: 5 -> [_]
                    tunnel: w695 -> [w715]
                    tunnel: w690 -> [w711]
                    tunnel: w694 -> [w710]
                    tunnel: [w709] -> w693
                    i -> [w713]
                    n390 = Add(x=w713, y=86) -> (x+y=w714:i32)
                    n391 = property class="Tree (严格)"(reference=w715, error in=w710, "Active Item Row Number"=w714, "Disabled?"=w711) -> (error out=w709:errorcluster)  [unwired: 1 out]
                  }
                  n392 = property on="模块软件版本 2" class="MCListbox (严格)"("Visible"=w679) -> ()  [unwired: 2 in, 2 out]
                  n393 = property on="模块软件版本" class="Enum (严格)"("Visible"=w679) -> ()  [unwired: 2 in, 2 out]
                  n394 = property on="平台软件版本号" class="Str"("Visible"=w679) -> ()  [unwired: 2 in, 2 out]
                  n395 = property on="模块版本读取" class="Bool (严格)"("Visible"=w679) -> ()  [unwired: 2 in, 2 out]
                  n396 = property on="平台软件版本读取" class="Bool (严格)"("Visible"=w679) -> ()  [unwired: 2 in, 2 out]
                  n397 = call <vilib>:"Clear Errors.vi"("error in (no error)"=w693) -> ()  [unwired: 6 in, 1 out]
                }
                frame #1 {
                  n398 = global read "功能码全局.vi" "主板项目信息7"() -> (w755:bool[])
                  n399 = global read "功能码全局.vi" "主板控制类信息10"() -> (w751:bool[])
                  n400 = global read "功能码全局.vi" "主板故障阀值9"() -> (w754:bool[])
                  n401 = global read "功能码全局.vi" "主板项目信息4"() -> (w733:bool[])
                  n402 = global read "功能码全局.vi" "主板项目信息5"() -> (w742:bool[])
                  n403 = global read "功能码全局.vi" "主板项目信息6"() -> (w732:bool[])
                  n404 = global read "功能码全局.vi" "主板版本号11"() -> (w741:bool[])
                  n405 = Delete From Array(array=w732, length=1 ("长度"), index=0 ("索引")) -> (deleted portion=w743:bool[], array with subset deleted=w759:bool[])
                  n406 = Index Array(array=w733, index #1=5 ("索引"), index #2=6 ("索引"), index #3=7 ("索引")) -> (element #1=w744:bool, element #2=w760:bool, element #3=w716:bool)
                  n407 = Index Array(array=w741) -> (element #1=w748:bool, element #2=w764:bool)  [unwired: 2 in]
                  n408 = Array Subset(array=w754, index=2 ("索引"), length=3 ("长度")) -> (w746:bool[])
                  n409 = Delete From Array(array=w755, length=3 ("索引"), index=2 ("长度")) -> (deleted portion=w745:bool[], array with subset deleted=w761:bool[])
                  n410 = Array Subset(array=w751, index=4 ("索引"), length=2 ("长度")) -> (w747:bool[])
                  n411 = global read "功能码全局.vi" "18"() -> (w724:bool[])
                  n412 = global read "功能码全局.vi" "16"() -> (w725:bool[])
                  n413 = Insert Into Array(array=w742, new element #1=w743, new element #2=w744, new element #3=w745, new element #4=w746, new element #5=w747, new element #6=w748) -> (w765:bool[])  [unwired: 1 in]
                  n414 = Array Subset(array=w751, index=6 ("索引"), length=2 ("长度")) -> (w763:bool[])
                  n415 = Array Subset(array=w754, index=5 ("索引"), length=3 ("长度")) -> (w762:bool[])
                  n416 = And Array Elements(Boolean array=w765) -> (logical AND=w730:bool)
                  n417 = Array Subset(array=w724, index=0 ("索引"), length=8 ("长度")) -> (w722:bool[])
                  n418 = Array Subset(array=w725, index=4 ("索引"), length=4 ("长度")) -> (w721:bool[])
                  n419 = Or Array Elements(Boolean array=w765) -> (logical OR=w717:bool)
                  n420 = Insert Into Array(array=w759, new element #1=w760, new element #2=w761, new element #3=w762, new element #4=w763, new element #5=w764) -> (w766:bool[])  [unwired: 1 in]
                  n421 = property on="全部读取" class="Bool (严格)"("Visible"=w730) -> ()  [unwired: 2 in, 2 out]
                  n422 = global read "功能码全局.vi" "15"() -> (w723:bool[])
                  n423 = And Array Elements(Boolean array=w766) -> (logical AND=w731:bool)
                  n424 = property on="全部写入" class="Bool (严格)"("Visible"=w731) -> ()  [unwired: 2 in, 2 out]
                  n425 = Or Array Elements(Boolean array=w766) -> (logical OR=w767:bool)
                  n426 = Insert Into Array(array=w723, new element #1=w722, new element #2=w721) -> (w720:bool[])  [unwired: 1 in]
                  n427 = Or Array Elements(Boolean array=w720) -> (logical OR=w719:bool)
                  n428 = Compound Arithmetic op=OR(w716, w717, w767, w719) -> (w768:bool)
                  n429 = case shown="真" w768 {
                    frame False {
                    }
                    frame True {
                      n430 = local write "主界面选项"(enum32{"单选选项1", "单选选项2", "单选选项2 2", "单选选项2 3"}."单选选项1" ("主界面选项")) -> ()
                      n431 = local write "面板选择"(enum32{"读写参数", "版本读取", "其它诊断"}."读写参数" ("选项卡控件 2")) -> ()
                    }
                  }
                  n432 = property on="单选选项1" class="Bool (严格)"("Visible"=w768) -> ()  [unwired: 2 in, 2 out]
                }
                frame #2 {
                  n433 = control-ref of="单选选项2 2"() -> (w775:refnum<vi>)
                  n434 = control-ref of="单选选项2 3"() -> (w771:refnum<vi>)
                  n435 = control-ref of="单选选项2"() -> (w777:refnum<vi>)
                  n436 = control-ref of="单选选项1"() -> (w776:refnum<vi>)
                  n437 = local read "主界面选项"() -> (w780:enum32{"单选选项1", "单选选项2", "单选选项2 2", "单选选项2 3"})
                  n438 = Build Array(w776, w777, w775, w771) -> (w774:refnum<vi>[])
                  n439 = Delete From Array(array=w774, index=w780) -> (deleted portion=w778:refnum<vi>, array with subset deleted=w779:refnum<vi>[])  [unwired: 1 in]
                  n440 = property class="Bool (严格)"(reference=w778, "BoolText.TextColor"=u32 87470) -> ()  [unwired: 1 in, 2 out]
                  n441 = for {
                    tunnel: u32 16777215 -> [w782]
                    tunnel: w779 -> [w781] mode=indexing
                    n442 = property class="Bool (严格)"(reference=w781, "BoolText.TextColor"=w782) -> ()  [unwired: 1 in, 2 out]
                  }
                }
              }
            }
            frame #1 {
              # "项目信息"
              # "SOC"
              # "SOH"
              # "电池额定实际容量"
              # "车牌号"
              # "产品编号"
              # "电压个数"
              # "通道电压数"
              # "温度个数"
              # "电压起始值"
              # "温度起始值"
              # "配置文件版本"
              # "系统时钟"
              # "校正时钟"
              n443 = global read "功能码全局.vi" "主板项目信息5"() -> (w856:bool[])
              n444 = global read "功能码全局.vi" "主板项目信息6"() -> (w855:bool[])
              n445 = global read "功能码全局.vi" "主板项目信息7"() -> (w832:bool[])
              n446 = global read "功能码全局.vi" "主板项目信息4"() -> (w803:bool[])
              n447 = Index Array(array=w856) -> (element #1=w853:bool, element #2=w850:bool, element #3=w847:bool, element #4=w844:bool, element #5=w840:bool, element #6=w838:bool, element #7=w835:bool, element #8=w831:bool)  [unwired: 8 in]
              n448 = Index Array(array=w855) -> (element #1=w828:bool, element #2=w852:bool, element #3=w849:bool, element #4=w846:bool, element #5=w843:bool, element #6=w839:bool, element #7=w837:bool, element #8=w834:bool)  [unwired: 8 in]
              n449 = Index Array(array=w832) -> (element #1=w830:bool, element #2=w827:bool, element #3=w825:bool, element #4=w820:bool, element #5=w817:bool, element #6=w824:bool, element #7=w818:bool, element #8=w816:bool)  [unwired: 8 in]
              n450 = Index Array(array=w803) -> (element #6=w799:bool, element #7=w798:bool, element #8=w802:bool)  [unwired: 8 in, 5 out]
              n451 = Not(x=w802) -> (.not. x?=w801:bool)
              n452 = Not Or(1:w798, 2:w799) -> (0:w797:bool)
              n453 = Not Or(1:w852, 2:w853) -> (0:w815:bool)
              n454 = Not Or(1:w849, 2:w850) -> (0:w814:bool)
              n455 = Not Or(1:w846, 2:w847) -> (0:w813:bool)
              n456 = Not Or(1:w843, 2:w844) -> (0:w812:bool)
              n457 = Not Or(1:w839, 2:w840) -> (0:w811:bool)
              n458 = Not Or(1:w837, 2:w838) -> (0:w810:bool)
              n459 = Not Or(1:w834, 2:w835) -> (0:w809:bool)
              n460 = Not Or(1:w830, 2:w831) -> (0:w808:bool)
              n461 = Not Or(1:w824, 2:w825) -> (0:w806:bool)
              n462 = Not Or(1:w816, 2:w817) -> (0:w804:bool)
              n463 = Not Or(1:w818, 2:w820) -> (0:w805:bool)
              n464 = Not Or(1:w827, 2:w828) -> (0:w807:bool)
              n465 = Compound Arithmetic op=OR(w801, w815, w814, w813, w812, w811, w810, w809, w808, w807, w806, w805, w804) -> (w796:bool)
              "项目信息结果" <- w796
              n466 = property class="Tree (严格)"(reference=w823, "Active Item Row Number"=9 ("活动项:行数"), "Disabled?"=w797, "Active Item Row Number"=1 ("活动项:行数"), "Disabled?"=w796, "Active Item Row Number"=0 ("活动项:行数"), "Disabled?"=w801, "Active Item Row Number"=3 ("活动项:行数"), "Disabled?"=w815, "Active Item Row Number"=4 ("活动项:行数"), "Disabled?"=w814, "Active Item Row Number"=5 ("活动项:行数"), "Disabled?"=w813, "Active Item Row Number"=6 ("活动项:行数"), "Disabled?"=w812, "Active Item Row Number"=7 ("活动项:行数"), "Disabled?"=w811, "Active Item Row Number"=8 ("活动项:行数"), "Disabled?"=w810, "Active Item Row Number"=11 ("活动项:行数"), "Disabled?"=w809, "Active Item Row Number"=12 ("活动项:行数"), "Disabled?"=w808, "Active Item Row Number"=13 ("活动项:行数"), "Disabled?"=w807, "Active Item Row Number"=2 ("活动项:行数"), "Disabled?"=w806, "Active Item Row Number"=10 ("活动项:行数"), "Disabled?"=w805, "Active Item Row Number"=14 ("活动项:行数"), "Disabled?"=w804) -> ()  [unwired: 1 in, 2 out]
            }
            frame #2 {
              w866 = 18
              # "一二三级故障"
              n467 = global read "功能码全局.vi" "主板故障阀值9"() -> (w872:bool[])
              n468 = Index Array(array=w872) -> (element #3=w871:bool, element #4=w868:bool, element #5=w865:bool, element #6=w870:bool, element #7=w867:bool, element #8=w864:bool)  [unwired: 8 in, 2 out]
              n469 = Not Or(1:w870, 2:w871) -> (0:w860:bool)
              n470 = Not Or(1:w867, 2:w868) -> (0:w858:bool)
              n471 = Not Or(1:w864, 2:w865) -> (0:w859:bool)
              n472 = for {
                N: w866 -> [_]
                tunnel: w861 -> [w892]
                tunnel: w860 -> [w888]
                tunnel: [w887] -> w869
                i -> [w890]
                n473 = Add(x=w890, y=15) -> (x+y=w891:i32)
                n474 = property class="Tree (严格)"(reference=w892, "Active Item Row Number"=w891, "Disabled?"=w888) -> (error out=w887:errorcluster)  [unwired: 1 in, 1 out]
              }
              n475 = for {
                N: w866 -> [_]
                tunnel: w861 -> [w886]
                tunnel: w858 -> [w882]
                tunnel: w869 -> [w881]
                tunnel: [w880] -> w863
                i -> [w884]
                n476 = Add(x=w884, y=33) -> (x+y=w885:i32)
                n477 = property class="Tree (严格)"(reference=w886, error in=w881, "Active Item Row Number"=w885, "Disabled?"=w882) -> (error out=w880:errorcluster)  [unwired: 1 out]
              }
              n478 = for {
                N: w866 -> [_]
                tunnel: w861 -> [w879]
                tunnel: w859 -> [w875]
                tunnel: w863 -> [w874]
                tunnel: [w873] -> w862
                i -> [w877]
                n479 = Add(x=w877, y=51) -> (x+y=w878:i32)
                n480 = property class="Tree (严格)"(reference=w879, error in=w874, "Active Item Row Number"=w878, "Disabled?"=w875) -> (error out=w873:errorcluster)  [unwired: 1 out]
              }
              n481 = call <vilib>:"Clear Errors.vi"("error in (no error)"=w862) -> ()  [unwired: 6 in, 1 out]
            }
          }
        }
        frame Enabled {
        }
      }
      n482 = disable-structure shown="禁用" {
        disable-tunnel: [w545 _] -> w544
        frame Disabled {
          n483 = control-ref of="从板选项"() -> (w546:refnum<vi>)
          n484 = stacked-sequence {
            tunnel: w546 -> [w549 w586 w628]
            tunnel: [w547 _ _] -> w545
            frame #0 {
